vi "FromRepo.vi"(8 "error in":errorcluster, 9 "cluster":T2, 10 "repository in":refnum<class "NISE_CEF_Repository.lvclass">, 11 "cRIO in":refnum<class "can port.lvclass">) -> (0 "error out":errorcluster, 2 "repository out":refnum<class "NISE_CEF_Repository.lvclass">, 3 "node":T1)   [LabVIEW 2013, in "can port.lvclass"]
uses:
  can port.lvclass
  <vilib>/NI/Configuration Framework/Repository/NISE_CEF_Repository.lvclass
  <vilib>/NI/Configuration Framework/Node/FromRepoCluster.ctl
  <vilib>/NI/Configuration Framework/Node/NodeRef.ctl
  <vilib>/NI/Configuration Framework/Node/NISE_CEF_Node.lvclass
  database file/database file.lvclass
  database file/database file.lvclass/database file.ctl
  can port.lvclass/can port.ctl
  database file/Read BaudRate.vi
  database file/Read J1939 Network Address.vi
  database file/Read Name.vi
  database file/Read frames.vi
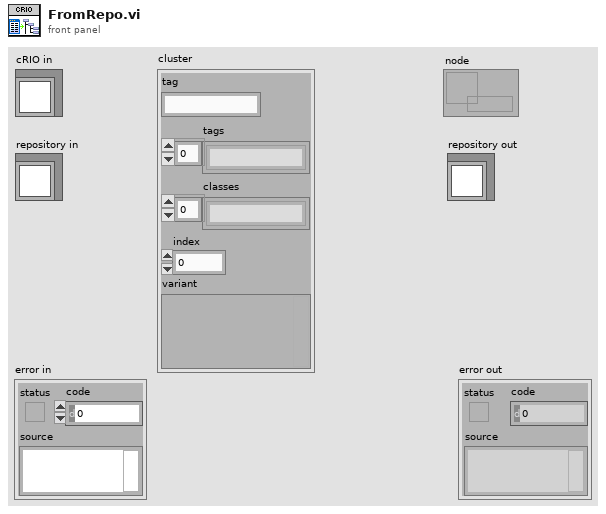
[diagram p1: front panel]
types:
  T1 = typedef "NISE_CEF_Node.lvclass/NodeRef.ctl" = refnum<data-value>
  T2 = typedef "NISE_CEF_Node.lvclass/FromRepoCluster.ctl" = cluster{"tag":string, "tags":string[], "classes":string[], "index":i32, "variant":variant}
  T3 = typedef "J1939.lvlib/J1939 db frame.ctl" = cluster{"name":string, "Priority":u8, "PGN":u32, "Reserved Bit":u8, "Data page":u8, "PDU Format":u8, "PDU Specific":u8, "Source Address":u8, "PayldLen":u32, "signals":T4[], "Comment":string, "can timing type":u32, "transmit time":dbl, "direction":u16}
  T4 = typedef "J1939.lvlib/J1939 db signal.ctl" = cluster{"NameShort":string, "SPN":i32, "StartBit":u32, "NumBits":u32, "DataType":u32, "ByteOrdr":u32, "ScaleFac":dbl, "ScaleOff":dbl, "Max":dbl, "Min":dbl, "Default":dbl, "Unit":string, "Comment":string}
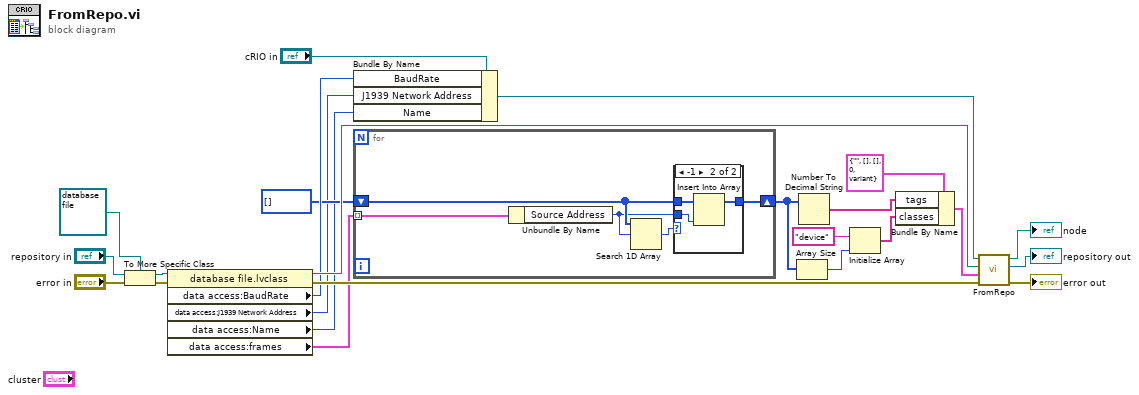
[diagram p0: block diagram]
diagram:
  n1 = To More Specific Class(target class=refnum<class "database file.lvclass"> refnum ("cRIO repo.lvclass"), reference="repository in", error in="error in") -> (specific class reference=w19:refnum<class "database file.lvclass">, error out=w16:errorcluster)
  n2 = property class="database file.lvclass"(reference=w19, error in=w16) -> (reference out=w18:refnum<class "database file.lvclass">, error out=w15:errorcluster, "data access:BaudRate"=w10:u32, "data access:J1939 Network Address"=w2:u8, "data access:Name"=w1:u64, "data access:frames"=w9:T3[])
  n3 = Bundle By Name(cluster="cRIO in", "BaudRate"=w10, "J1939 Network Address"=w2, "Name"=w1) -> (w11:refnum<class "can port.lvclass">)
  n4 = for {
    tunnel: w9 -> [w29] mode=indexing
    shift-right: [w27] -> w4
    shift-left: u8[] [] ("array in") -> [w28]
    n5 = Unbundle By Name(w29) -> ("Source Address"=w26:u8)
    n6 = Search 1D Array(1D array=w28, element=w26) -> (index of element=w25:i32)  [unwired: 1 in]
    n7 = case shown="-1" w25 {
      tunnel: [w30 w32] -> w27
      tunnel: w28 -> [w30 w33]
      tunnel: w26 -> [_ w31]
      frame 0, Default {
      }
      frame -1 {
        n8 = Insert Into Array(array=w33, new element=w31) -> (w32:u8[])  [unwired: 1 in]
      }
    }
  }
  n9 = Array Size(array=w4) -> (size(s)=w6:i32)
  n10 = Number To Decimal String(number=w4) -> (decimal integer string=w3:string[])  [unwired: 1 in]
  n11 = Initialize Array("device" ("Tag"), w6) -> (w5:string[])
  n12 = Bundle By Name(cluster=T2 {"tag"="", "tags"=[], "classes"=[], "index"=0, "variant"=variant} ("Cluster"), "tags"=w3, "classes"=w5) -> (w13:T2)
  n13 = call-parent "FromRepo.vi"("error in"=w15, "from repo cluster"=w13, "repository in"=w18, "node in"=w11) -> ("error out"=→"error out":errorcluster, "repository out"=→"repository out":refnum<class "NISE_CEF_Repository.lvclass">, "node"=→"node":T1)  [unwired: 5 in]
